vi "N Channel 1 Sample - Manual Timestamp.vi"() -> ()   [LabVIEW 2026, in "synnax_clib.lvlib"]
uses:
  lvlib/synnax_clib.lvlib
  lvlib/typedefs/connection_config.ctl
  lvlib/classes/Client/Private/synnax channel retrieve keys Array.vi
  lvlib/classes/Writer/Private/synnax writer open Array.vi
  lvlib/classes/Writer/Private/Writes/I32/Write NCh 1Samp (I32).vi
  lvlib/classes/Synnax Writer.lvclass
  lvlib/classes/Client/Synnax Client.lvclass
panel:
  out "error out":errorcluster
  in  "Channels":string[](array[numeric])=["my_i32_idx", "my_i32_ch1", "my_i32_ch2", "my_i32_ch3", "my_i32_ch4"]
  in  "Stop":bool
  in  "Connection Config":T1={"host"="localhost", "port"=9090, "username"="synnax", "password"="seldon"}
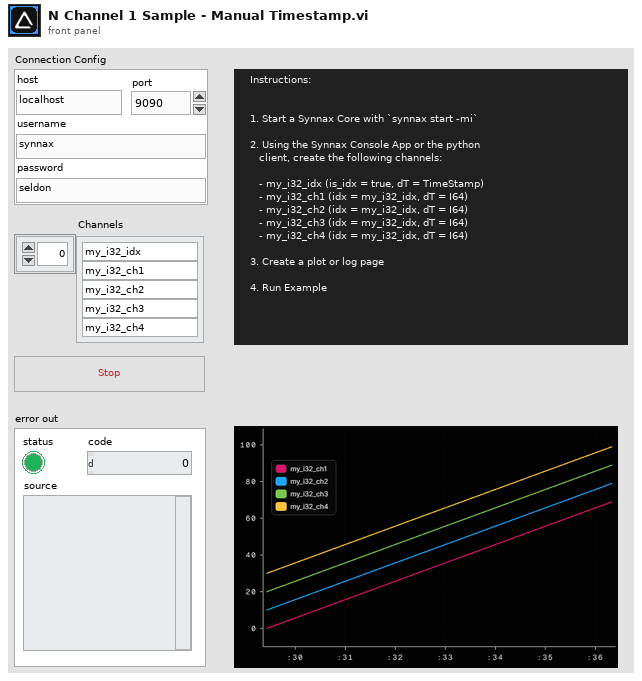
[diagram p1: front panel]
types:
  T1 = typedef "synnax_clib.lvlib/connection_config.ctl" = cluster{"host":string, "port":u16, "username":string, "password":string}
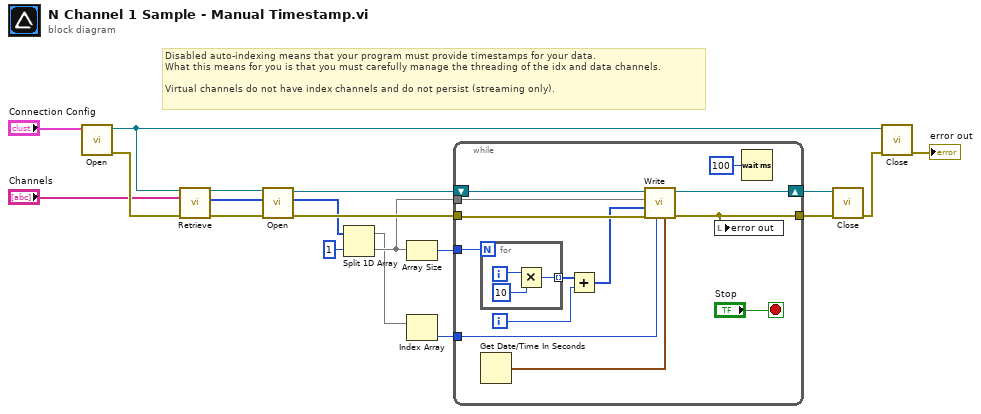
[diagram p0: block diagram]
diagram:
  # "Disabled auto-indexing means that your program must provide timestamps for your data.\nWhat this means for you is that you must carefully manage the threading of the idx and data channels.\n\nVirtual channels do not have index channels and do not persist (streaming only)."
  n1 = call "Open.vi"("Connection Config"="Connection Config") -> ("error out"=w14:errorcluster, "Synnax Client out"=w16:refnum<class "Synnax Client.lvclass">)  [unwired: 9 in]
  n2 = call-poly "Retrieve.vi"("Synnax Client in"=w16, "channel names"="Channels", "error in"=w14) -> ("Synnax Client out"=w10:refnum<class "Synnax Client.lvclass">, "channel keys"=w9:u32[], "error out"=w18:errorcluster)  [unwired: 8 in, 2 out]
  n3 = call-poly "Open.vi"("error in"=w18, "channels in"=w9, "Synnax Client in"=w10) -> ("error out"=w11:errorcluster, "channels out"=w7:u32[], "writer out"=w13:refnum<class "Synnax Writer.lvclass">)  [unwired: 6 in]
  n4 = Split 1D Array(array=w7, index=1) -> (first subarray=w3:u32[], second subarray=w5:u32[])
  n5 = Array Size(array=w5) -> (size(s)=w4:i32)
  n6 = Index Array(array=w3) -> (element=w2:u32)  [unwired: 1 in]
  n7 = while {
    shift-right: [w31] -> w12
    shift-left: w13 -> [w32]
    tunnel: w11 -> [w30]
    tunnel: [w27] -> w19
    tunnel: w5 -> [w25]
    tunnel: w4 -> [w24]
    tunnel: w2 -> [w21]
    i -> [w22]
    stop <- "Stop" stop-if-true
    n8 = for {
      N: w24 -> [_]
      tunnel: [w34] -> w28 mode=indexing
      i -> [w35]
      n9 = Multiply(x=w35, y=10) -> (x*y=w34:i32)
    }
    n10 = Get Date/Time In Seconds() -> (seconds since 1Jan1904=w20:timestamp)
    n11 = Add(x=w28, y=w22) -> (x+y=w23:i32[])
    n12 = call-poly "Write.vi"("timestamp"=w20, "index_channel"=w21, "error in"=w30, "data"=w23, "channels"=w25, "Writer"=w32) -> ("error out"=w27:errorcluster, "Writer Out"=w31:refnum<class "Synnax Writer.lvclass">)  [unwired: 4 in]
    n13 = local write "error out"(w27) -> ()
    n14 = Wait (ms)(milliseconds to wait=u32 100) -> ()  [unwired: 1 out]
  }
  n15 = call "Close.vi"("error in"=w19, "writer"=w12) -> ("error out"=w15:errorcluster)  [unwired: 9 in]
  n16 = call "Close.vi"("error in"=w15, "Synnax Client in"=w16) -> ("error out"=→"error out":errorcluster)  [unwired: 9 in]
